vi "scantimingsource_1ms_10dt.vi"() -> (0 "max jitter (uS)":dbl format="%.2f", 1 "mean time (uS)":dbl format="%.2f", 2 "standard deviation (uS)":dbl format="%.2f", 3 "execution histogram":T1(graph), 4 "Error":errorcluster, 5 "execution times (uS)":dbl[](graph))   [LabVIEW 2013]
uses:
  <vilib>/Platform/TimedLoop/XDataNode/timing_clust.ctl
  <vilib>/Platform/TimedLoop/XDataNode/nitl_modes.ctl
  <vilib>/Platform/TimedLoop/XDataNode/wakeup.ctl
  <vilib>/Platform/TimedLoop/XDataNode/loadnilvce.vi
  <vilib>/platform/TimedLoop/XDataNode/XDataNode.xnode
  <vilib>/Platform/TimedLoop/XDataNode/XDNodeRunTimeDep.lvlib
  <vilib>/NI_Real-Time Target Support.lvlib
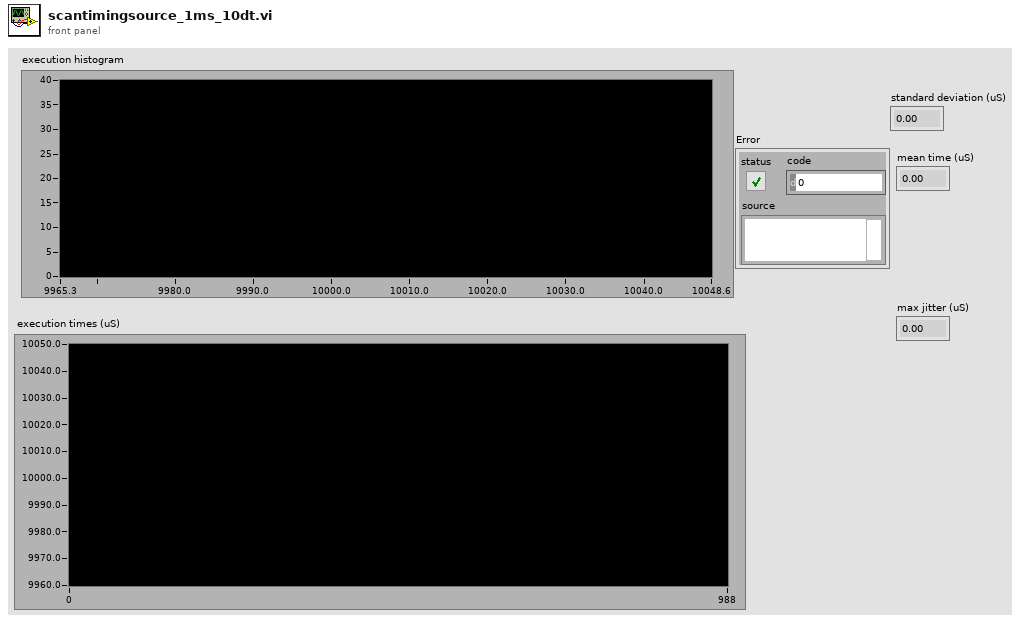
[diagram p1: front panel]
types:
  T1 = cluster{"X Values":dbl[], "Histogram: h(x)":i32[]}
  T2 = typedef "XDNodeRunTimeDep.lvlib/timing_clust.ctl" = cluster{"Expected End [f-1]":u64, "Actual End [f-1]":u64, "Finished Late? [f-1]":bool, "Expected End [i-1]":u64, "Actual End [i-1]":u64, "Finished Late? [i-1]":bool, "Expected Start [i]":u64, "Actual Start [i]":u64, "Expected Start [f]":u64, "Actual Start [f]":u64, "Source Name":string, "Structure Name":string, "Period":i64, "Deadline":i64, "Offset":i64, "Start":i64, "Priority":i32, "Timeout":i32, "Mode":T3, "Wakeup Reason":T4, "Error":errorcluster, "Source Type":string, "Secondary Source Type":string, "Global End Time":u64, "Global Start Time":u64, "Frame Duration":u64, "Iteration Duration":u64, "Assigned CPU":i32, "I/O Scan Engine Mode":u32}
  T3 = typedef "XDNodeRunTimeDep.lvlib/nitl_modes.ctl" = enum32{"No Change", "Process missed periods, maintain original phase", "Discard missed periods, maintain original phase", "Process missed periods, ignore original phase", "Discard missed periods, ignore original phase"}
  T4 = typedef "XDNodeRunTimeDep.lvlib/wakeup.ctl" = enum32{"Normal", "Aborted", "Asynchronous wakeup", "Timing source error", "Timed loop error", "Timeout"}
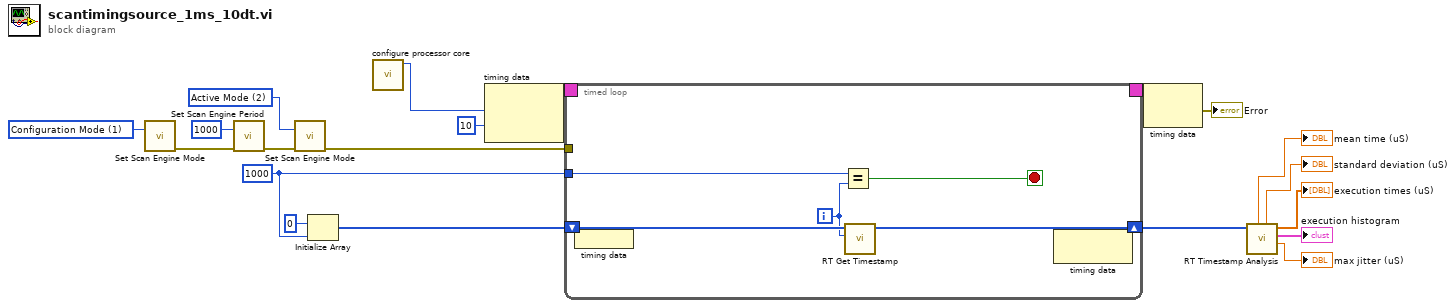
[diagram p0: block diagram]
diagram:
  w12 = 1000 ("x")
  w17 = 1 items=["Configuration Mode"=1, "Active Mode"=2] ("mode (Active Mode)")
  w18 = 2 items=["Configuration Mode"=1, "Active Mode"=2] ("mode (Active Mode)")
  n1 = call <vilib>:"Set Scan Engine Mode.vi"("mode (Active Mode)"=w17) -> ("error out"=w19:errorcluster)  [unwired: 14 in]
  n2 = call <vilib>:"Set Scan Engine Period.vi"("scan period (uSec)"=u32 1000, "error in (no error)"=w19) -> ("error out"=w20:errorcluster)  [unwired: 13 in]
  n3 = call <vilib>:"Set Scan Engine Mode.vi"("mode (Active Mode)"=w18, "error in (no error)"=w20) -> ("error out"=w15:errorcluster)  [unwired: 13 in]
  n4 = Initialize Array(u64 0, w12) -> (w13:u64[])
  n5 = call "configure processor core.vi"() -> ("Processor"=w1:i32)  [unwired: 11 in]
  n6 = node-c288(w1, i64 10 ("Period")) -> (w5:T2)
  n7 = timed-loop {
    timing: w5 -> [_]
    timing-out: [_] -> w4
    tunnel: w15 -> [_]
    shift-right: [w22] -> w11
    shift-left: w13 -> [w23]
    tunnel: w12 -> [w25]
    i -> [w21]
    stop <- w24 stop-if-true
    n8 = node-c288() -> ()  [unwired: 1 in]
    n9 = Equal?(x=w25, y=w21) -> (x = y?=w24:bool)
    n10 = call <vilib>:"RT Get Timestamp.vi"("iteration"=w21, "timestamp array in"=w23) -> ("timestamp array out"=w22:u64[])  [unwired: 8 in, 1 out]
    n11 = node-c288() -> ()  [unwired: 1 in, 1 out]
  }
  n12 = node-c288(w4) -> (→"Error":errorcluster)
  n13 = call <vilib>:"RT Timestamp Analysis.vi"("timestamp array"=w11) -> ("max jitter (uS)"=→"max jitter (uS)":dbl, "execution histogram"=→"execution histogram":T1, "execution times (uS)"=→"execution times (uS)":dbl[], "standard deviation (uS)"=→"standard deviation (uS)":dbl, "mean time (uS)"=→"mean time (uS)":dbl)  [unwired: 5 in, 1 out]
